vi "Keithley_run.vi"(0 "VISA Refnum in":refnum<visa-resource-name>, 1 "Meas. CH Type":T3 items=["Voltage", "Current", "IV"], 2 "Init timer":u32, 5 "Node Out":string, 7 "Input CH Type":T1 items=["Current", "Voltage", ""], 9 "Channel (Channel A)":T2, 11 "error constant":errorcluster, 12 "Final value":dbl, 13 "Initial value":dbl, 14 "Interval time":dbl) -> (3 "x+y":dbl, 4 "VISA Refnum out":refnum<visa-resource-name>, 6 "Node Out out":string, 8 "Boolean":bool, 10 "Output":string, 15 "error constant 2":errorcluster)   [LabVIEW 2012]
uses:
  controls/MeasurementType.ctl
  Keithley 2600 Series/Public/Channel.ctl
  Keithley 2600 Series/Keithley 2600 Series.lvlib
  controls/KeithlyChannelType.ctl
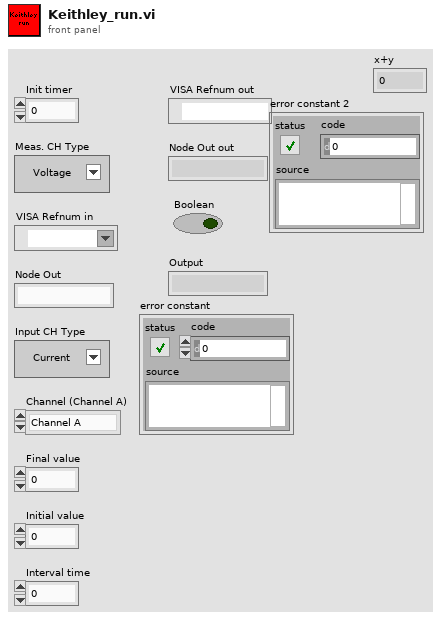
[diagram p1: front panel]
types:
  T1 = typedef "KeithlyChannelType.ctl" = u16
  T2 = typedef "Keithley 2600 Series.lvlib/Channel.ctl" = enum32{"Channel A", "Channel B"}
  T3 = typedef "MeasurementType.ctl" = u16
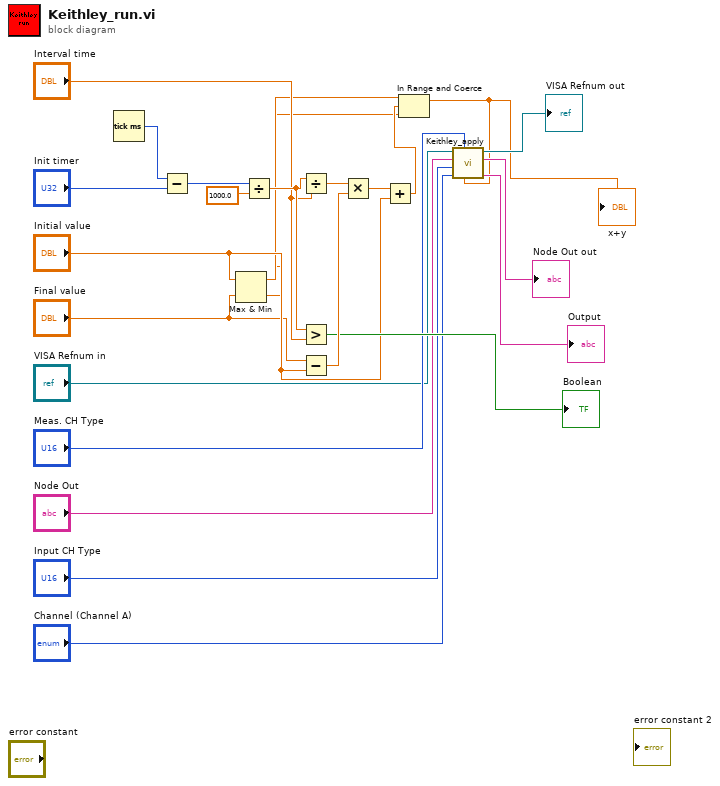
[diagram p0: block diagram]
diagram:
  n1 = Tick Count (ms)() -> (millisecond timer value=w17:u32)
  n2 = Subtract(x=w17, y="Init timer") -> (x-y=w20:u32)
  n3 = Max & Min(x="Initial value", y="Final value") -> (max(x,y)=w2:dbl, min(x,y)=w1:dbl)
  n4 = Divide(x=w20, y=1000.0) -> (x/y=w8:dbl)
  n5 = Divide(x=w8, y="Interval time") -> (x/y=w22:dbl)
  n6 = Greater?(x=w8, y="Interval time") -> (0:→"Boolean":bool)
  n7 = Subtract(x="Final value", y="Initial value") -> (x-y=w23:dbl)
  n8 = Multiply(x=w22, y=w23) -> (x*y=w24:dbl)
  n9 = Add(x=w24, y="Initial value") -> (x+y=w5:dbl)
  n10 = In Range and Coerce(upper limit=w2, x=w5, lower limit=w1) -> (coerced(x)=w6:dbl)  [unwired: 1 out]
  "x+y" <- w6
  n11 = call "Keithley_apply.vi"("Level"=w6, "Meas. CH Type"="Meas. CH Type", "Channel (Channel A)"="Channel (Channel A)", "Input CH Type"="Input CH Type", "Node Out in"="Node Out", "VISA Refnum in"="VISA Refnum in") -> ("Output"=→"Output":string, "Node Out out"=→"Node Out out":string, "VISA Refnum out"=→"VISA Refnum out":refnum<visa-resource-name>)  [unwired: 3 in]
